vi "uintDecimalStringToUint.vi"(8 "Error in (no error)":errorcluster, 9 "Base (decimal)":T1=10 items=["Binary"=2, "Octal"=8, "Decimal"=10, "Hexadecimal"=16, "Hexatrigesimal"=36, "ASCII"=64], 10 "String":string) -> (0 "Error out":errorcluster, 3 "Uint out":refnum<class "UintClass.lvclass">)   [LabVIEW 2011]
uses:
  UintClass.lvclass
  enumBase.ctl
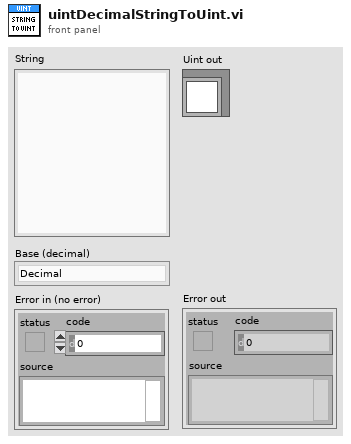
[diagram p1: front panel]
types:
  T1 = typedef "UintClass.lvclass/enumBase.ctl" = u16
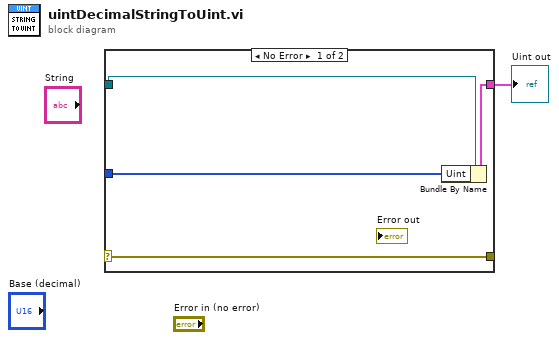
[diagram p0: block diagram]
diagram:
  n1 = case shown="No Error" w5 {
    selector: [w9 w10] -> w5
    tunnel: [w9 w10] -> w4
    tunnel: [w7 w11] -> w2
    tunnel: [w8 w11] -> w3
    tunnel: [w6 _] -> w1
    frame No Error {
      n2 = Bundle By Name(cluster=w8, "Uint"=w6) -> (w7:cluster{})
    }
    frame Error {
    }
  }
  "Uint out" <- w2
